vi "IETS_Tool_14_0805_bias_correct_neg_setpoints_ProbeStation.vi"() -> ()   [LabVIEW 2013]
doc: "I. Description:\nThis example demonstrates how to continuously acquire and generate data at the same time, synchronized with one another.\n\nII. Instructions for Running:\n1. Select the physical channel to correspond to where your signal is input on the DAQ device. Also, select the corresponding channel for where your signal is being generated.\n2. Enter the minimum and maximum voltage ranges.\nNote: For better accuracy try to match the input range to the expected voltage level of the measured signal.\n3. Set the sample rate of the acquisition.\nNote: The rate should be at least twice as fast as the maximum frequency component of the signal being acquired. \n6. Select the Rate for the generation\n7. Select what type of signal to generate and the amplitude.\nNote: This example requires two DMA channels to run. If your hardware does not support two DMA channels, you need to set the Data Transfer Mechanism property for the Analog Output Task to use \"Interrupts\". The Data Transfer Mechanism property is located in the DAQmx Channel Property hierarchy at:\n\nDAQmx Channel Property Node>>Analog Output>>General Properties>>Advanced>>Data Transfer and Memory>>Data Transfer Mechanism\n\nRefer to your device documentation to determine how many DMA channels are supported for your hardware.\n\nIII. Block Diagram Steps:\n1. Create an analog input voltage channel. Also, create an analog output voltage channel.\n2. Set the rate for the sample clock. Additionally, define the sample mode to be continuous. Also, set the sample clock rate for the signal generation.\n2a. Call the Get Terminal Name with Device Prefix VI. This will take a Task and a terminal and create a properly formatted device + terminal name to use as the source of the Trigger.\n3. Define the parameters for a Digital Edge Start Trigger. Set the Analog output to trigger off the AI Start Trigger. This is an internal trigger signal.\n4. Use the Basic Function Generator VI to create the signal to be generated.\n5. Call the Start VI to arm the two functions. Make sure the analog output is armed before the analog input. This will ensure both will start at the same time.\n6. Read the waveform data in a loop until the user hits the stop button or an error occurs. The Is Task Done? VI is used to check for errors in the Analog Output Task.\n7. Call the Clear VI to Clear the Task\n8. Use the popup dialog box to display an error if any.\n\nIV. I/O Connections Overview:\nMake sure your signal input/output terminals match the Physical Channel I/O controls."
uses:
  <vilib>/Utility/error.llb/DialogType.ctl
  <vilib>/DAQmx/write.llb/DAQmx Write (Analog 2D DBL NChan NSamp).vi
  <vilib>/DAQmx/read.llb/DAQmx Read (Analog 1D DBL NChan 1Samp).vi
  <vilib>/DAQmx/write.llb/DAQmx Write (Analog DBL 1Chan 1Samp).vi
  <vilib>/DAQmx/read.llb/DAQmx Read (Analog DBL 1Chan 1Samp).vi
  <vilib>/Analysis/baseanly.llb/Mean (DBL).vi
  <vilib>/DAQmx/write.llb/DAQmx Write (Analog 1D DBL NChan 1Samp).vi
  <vilib>/DAQmx/create/channels.llb/DAQmx Create Channel (AO-Voltage-Basic).vi
  <vilib>/DAQmx/create/channels.llb/DAQmx Create Channel (AI-Voltage-Basic).vi
  <vilib>/DAQmx/configure/timing.llb/DAQmx Timing (Sample Clock).vi
  <vilib>/DAQmx/configure/trigger.llb/DAQmx Start Trigger (Digital Edge).vi
  <vilib>/DAQmx/miscellaneous.llb/DAQmx Fill In Error Info.vi
  <vilib>/Utility/file.llb/Write To Spreadsheet File (DBL).vi
  pid/pid.llb/PID (DBL).vi
  pid/pid.llb/PID Output Rate Limiter (DBL).vi
  <vilib>/ptbypt/NI_PtbyPt.lvlib
  <resource>/objmgr/daqmx.rc
  <vilib>/Analysis/NI_AALBase.lvlib
panel:
  in  "Bias Offset Correct":dbl
  out "Bias Sweep":dbl[](graph)
  out "element":dbl
  out "mean":dbl format="%.6f"
  out "size(s)":i32
  out "Numeric":i32
  in  "PID":bool=TRUE caption="Step Z"
  in  "Tab Control":enum32{"PID Controller", "Tapping Controls"}(tab)=enum."Tapping Controls"
  in  "Proportional Gain":dbl=0.0001
  in  "Integral Gain":dbl=1e-07
  in  "Differential Gain":dbl=1e-05
  in  "Setpoint":dbl=0.1
  in  "Piezo Delta rate":dbl=1000.0
  in  "Min Current":dbl=0.002
  in  "Max Current":dbl=10.2
  in  "Ramp Rate":dbl=20.0
  in  "Make Contact":i32=1200
  in  "Break Contact":i32=500
  in  "Step Length":i32=100
  in  "Step Max":dbl=0.3
  in  "Step Min":dbl=0.05
  out "Tapping Stop":bool
  out "Case":i32
  in  "Contact Cycles":i32
  in  "Tapping":bool caption="Step Z"
  out "x/y":dbl
  out "Waveform Chart":dbl(graph)
  in  "Analog Ouyput 1":dbl(slide) min=-10.0 max=10.0 step=0.001 scale=-10.0..10.0
  in  "Manual Z":bool caption="Step Z"
  in  "Sweep Amplitude":dbl=1.0
  in  "Stop Sweep":bool
  out "Connections 2":string="AI0=Current\nAI1=Bias\nAI2=dI/dV\nAI3=d2I/dV2\nAI4=X-Axis\nAI5=Z-Axis\n"
  out "Connections":string="AO0=Bias\nAO1=Z-axis\nAO2=X-Axis\nAO3=NA"
  out "Save Indicator":bool
  in  "Z-Direction":bool caption="Step Z"
  in  "Update Bias":bool
  in  "Save IV":bool
  in  "Save Decay":bool
  in  "Sweep Bias":bool
  in  "Step Z":bool
  in  "Comment":string="Molecule=TP4\nGain=10nA\nBias Gain=div/1\nSweep Freq.=0.0008Hz\nRef. Bias=4mV\nRef. Freq=2.977kHz\nGain LIA1=2mV\nTC LIA1=1s\nGain LIA2=5mV\nTC LIA2=1s\nLIA1=EGG\nLIA2=SRS\nEGG is driving(possible 5mV offset)"
  in  "Filenumber":i32
  in  "DATA Filename":string="Data_"
  in  "Data Directory":path=path "E:/Research/Data"
  out "Current Decay":cluster{dbl[], dbl[]}(graph)
  out "d2I/dV2":cluster{dbl[], dbl[]}(graph)
  out "dI/dV":cluster{dbl[], dbl[]}(graph)
  out "IV":cluster{dbl[], dbl[]}(graph)
  in  "# Samples":i32=2000
  in  "Frequency (Hz)":dbl=1.0
  out "Measurement 2":cluster{i32, dbl, dbl[]}(graph) caption="Measurement"
  out "Actual Update Generation Rate 2":dbl=5000.0 caption="Actual Update Generation Rate" format="%0.2f"
  in  "stop 3":bool
  in  "Bias":dbl=0.1 caption="Bias Start Point" step=0.1 format="%_3g"
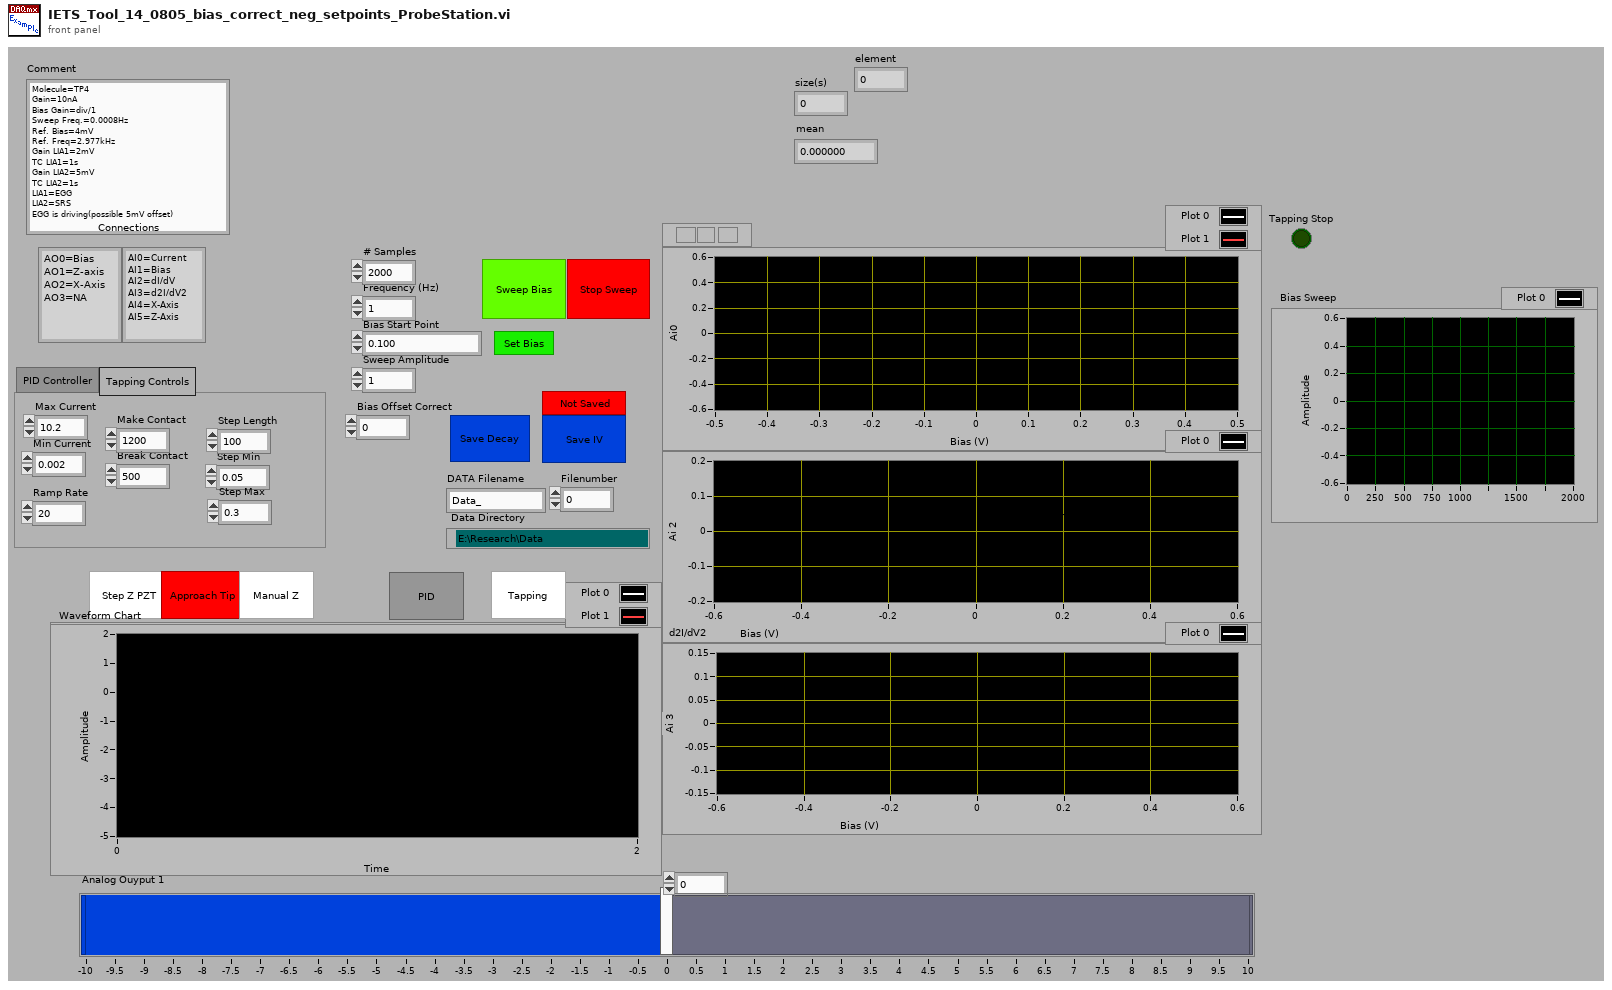
[diagram p1: front panel]
types:
  T1 = enum16{"open", "replace", "create", "open or create", "replace or create", "replace or create with confirmation"}
  T2 = typedef "DialogType.ctl" = u16
  T3 = cluster{"Proportional Gain":dbl, "Integral Gain ":dbl, "Differential Gain":dbl}
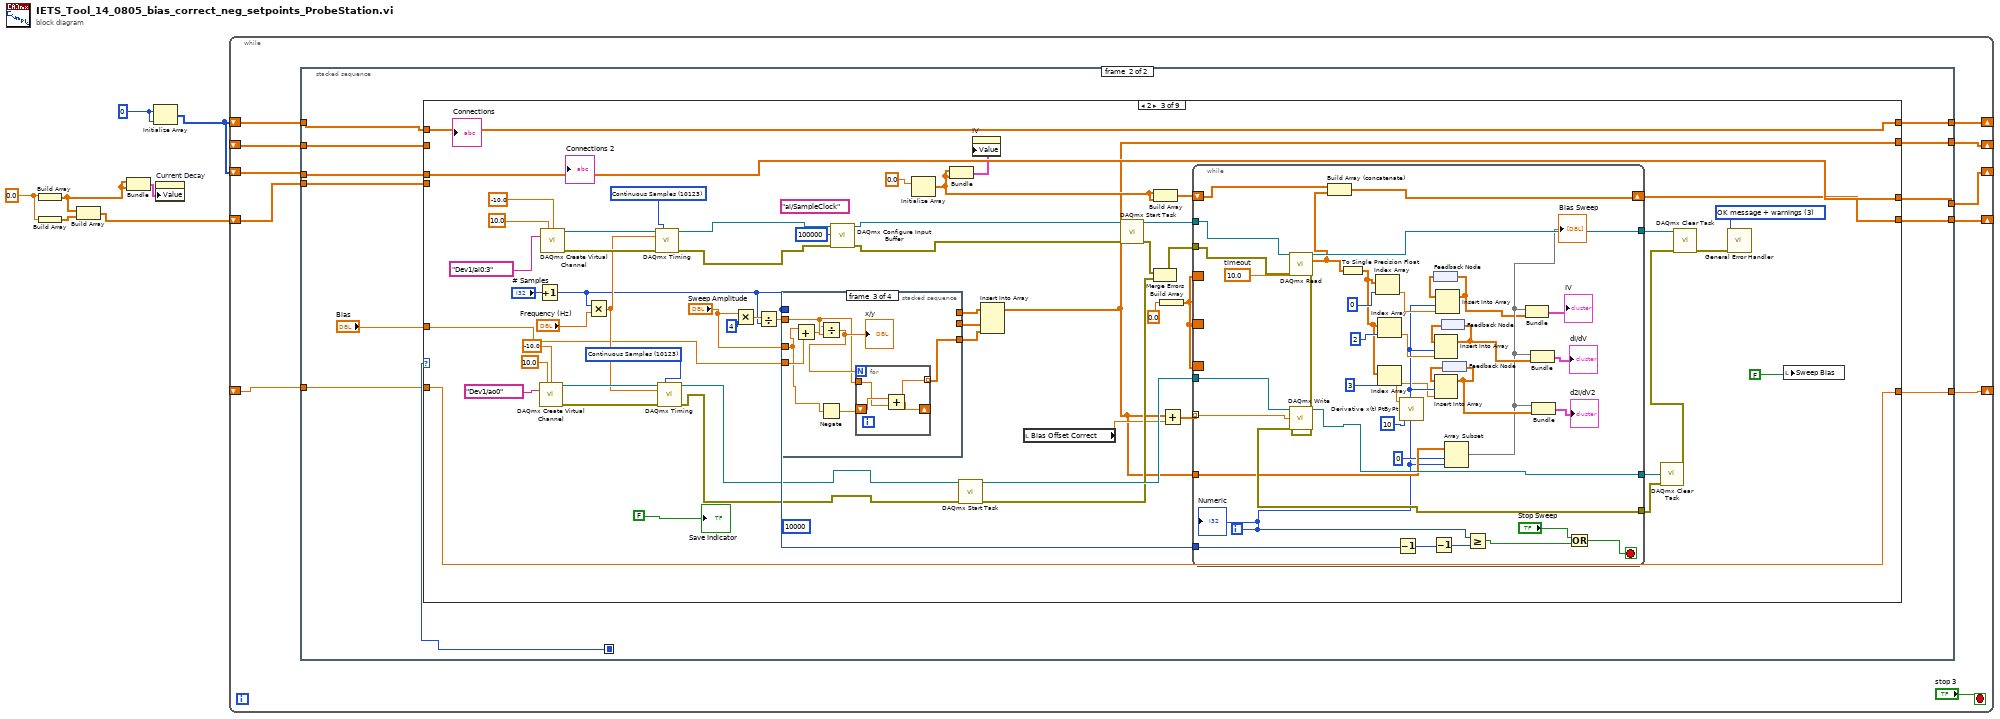
[diagram p0: block diagram]
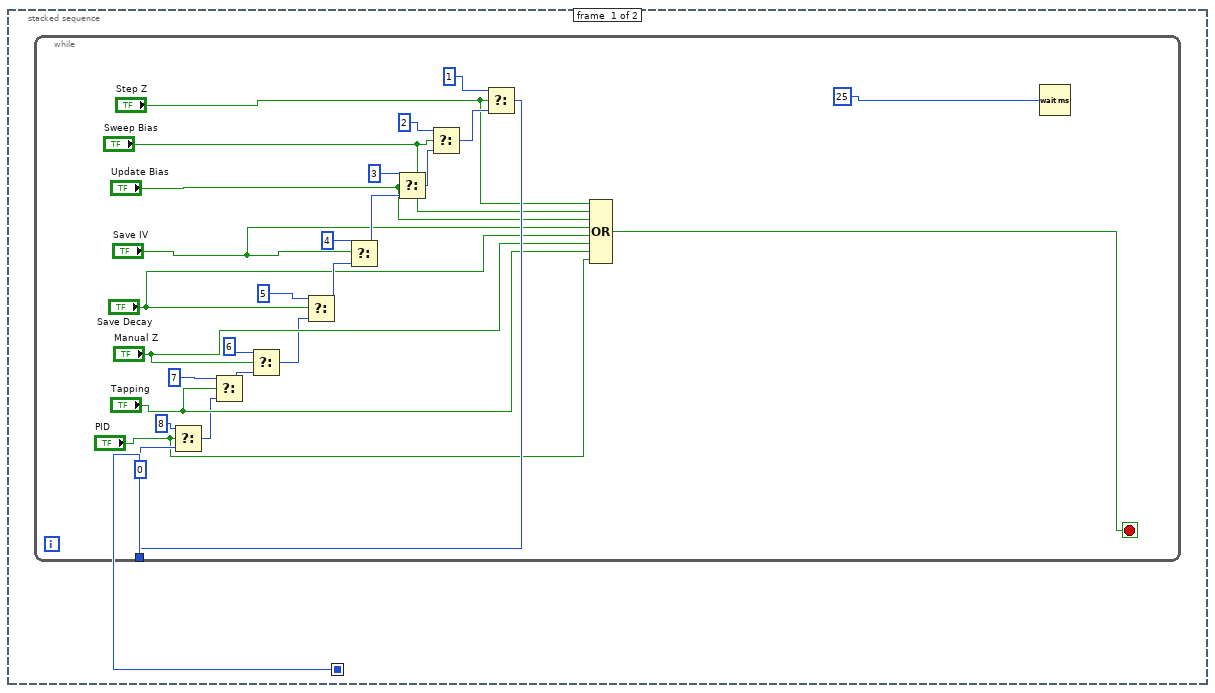
[diagram p2: hidden frame]
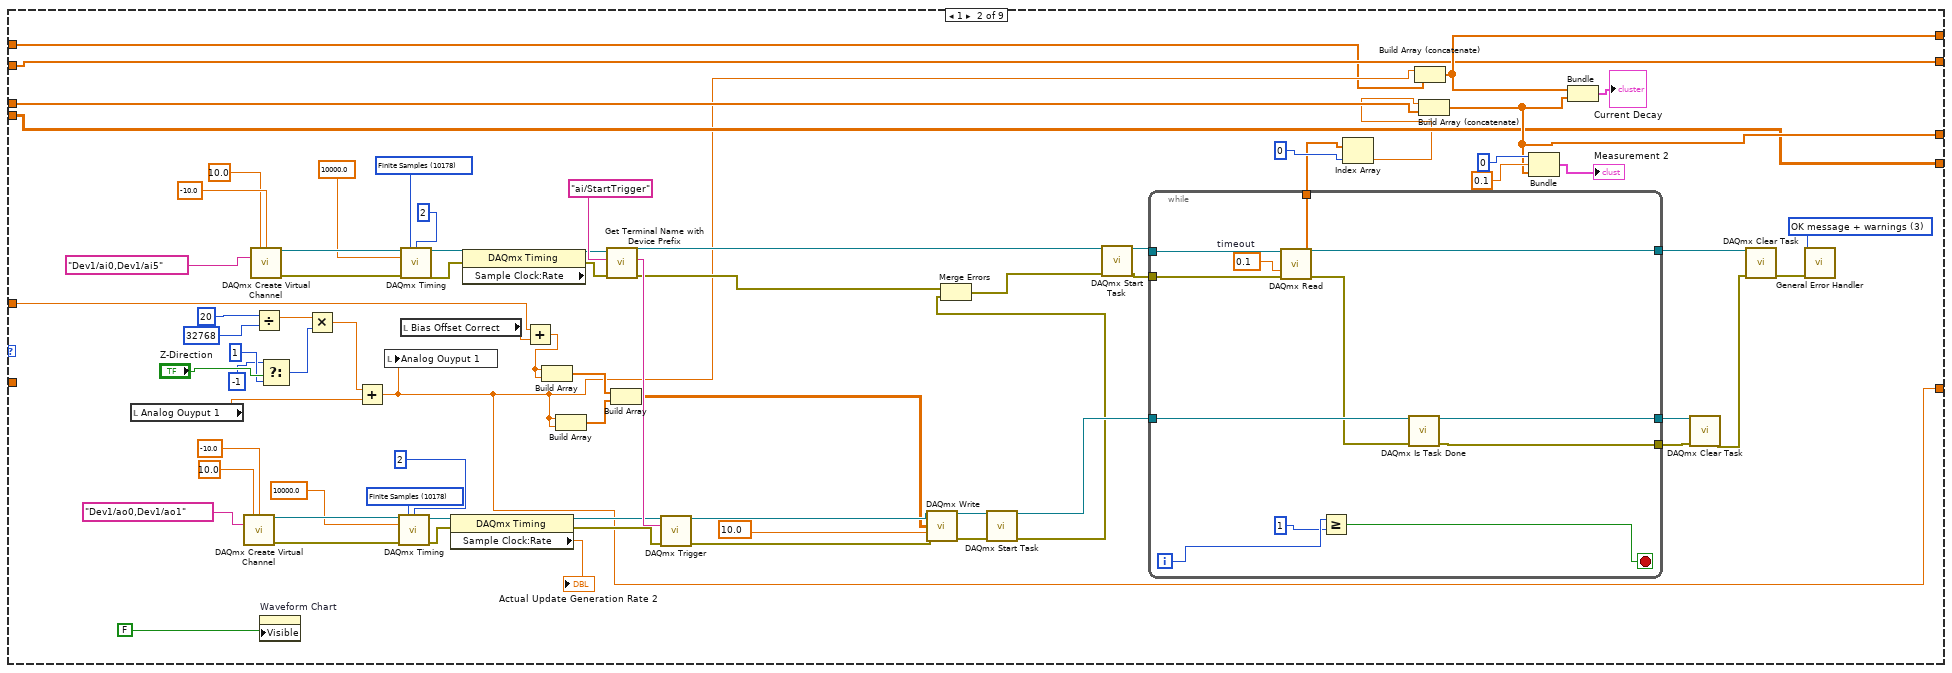
[diagram p4: hidden frame]
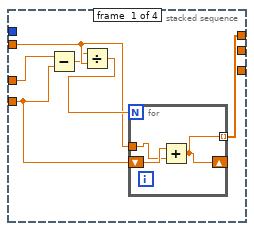
[diagram p5: hidden frame]
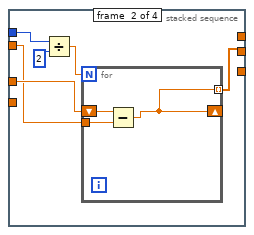
[diagram p6: hidden frame]
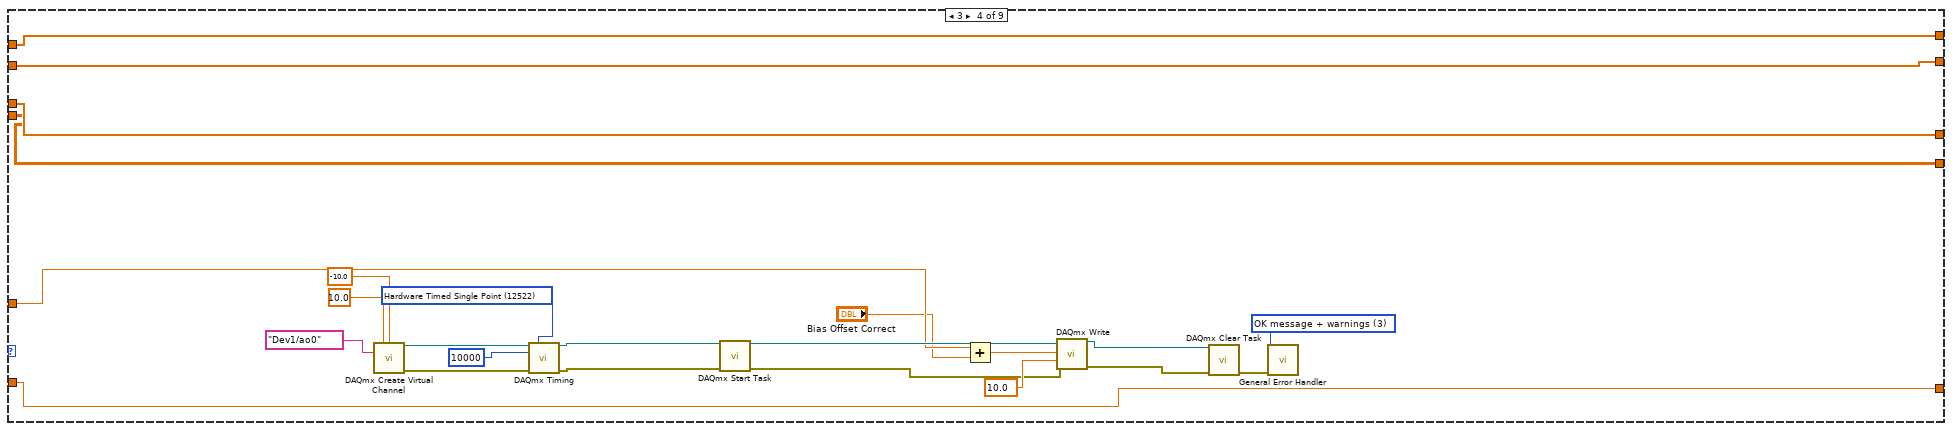
[diagram p8: hidden frame]
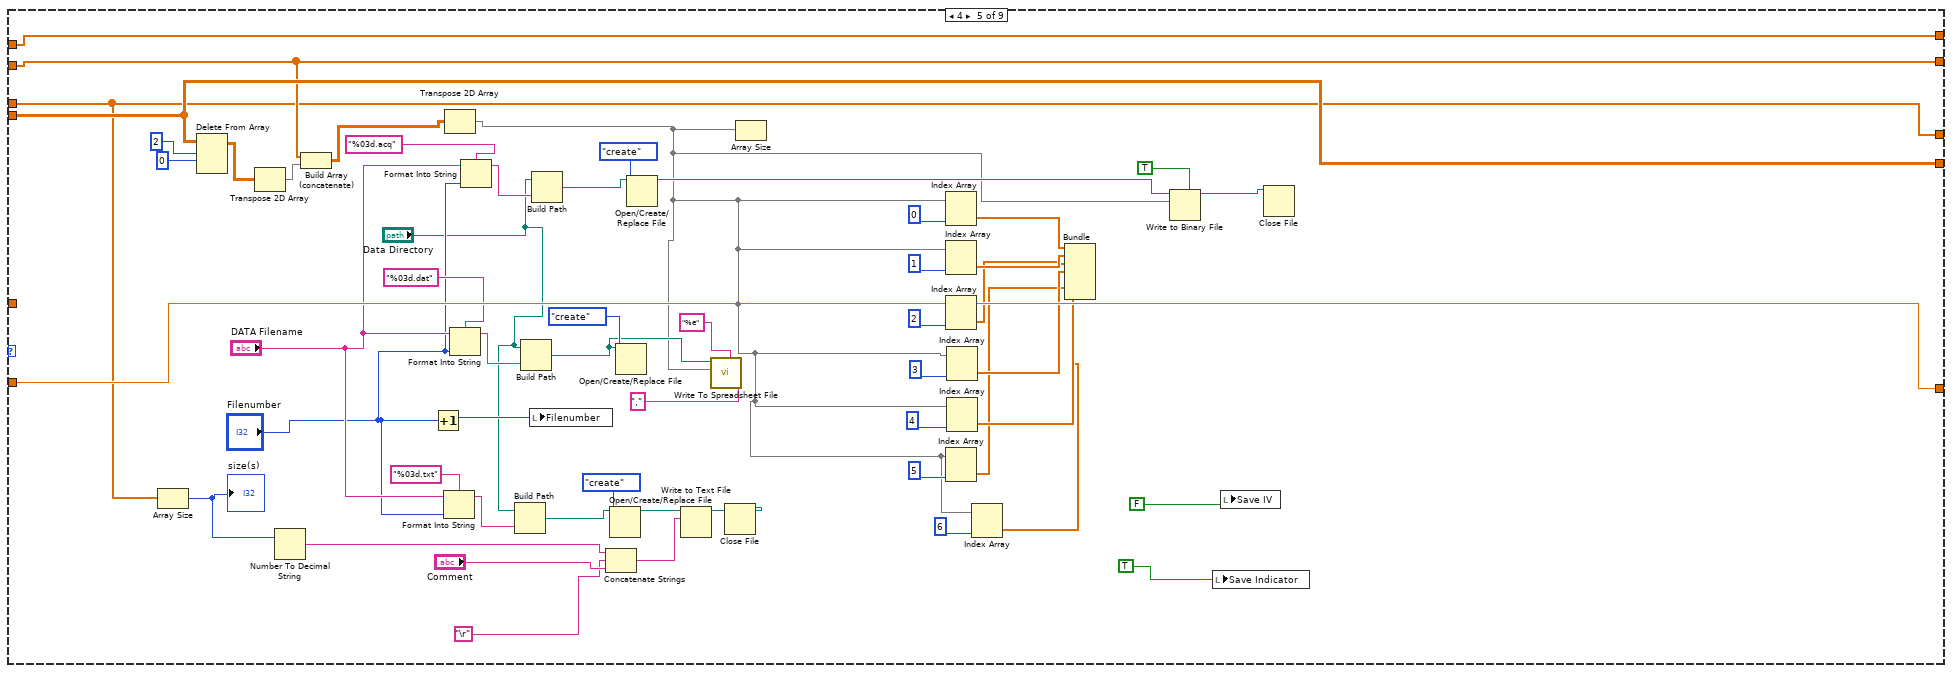
[diagram p9: hidden frame]
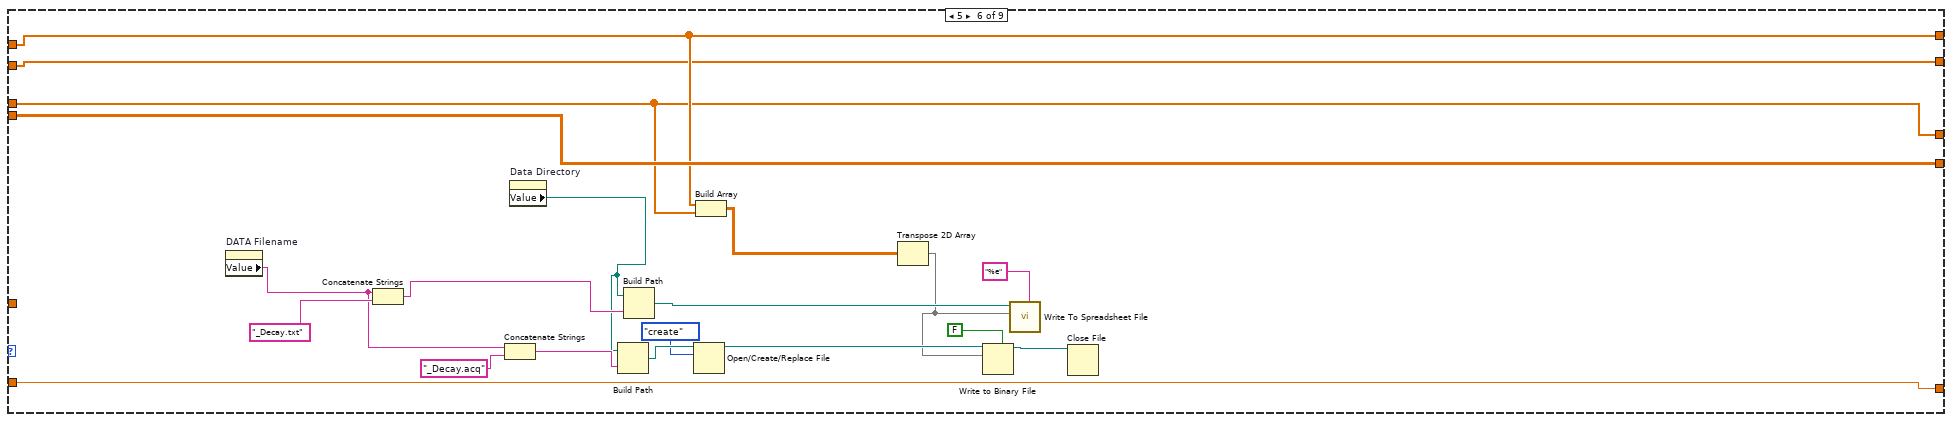
[diagram p10: hidden frame]
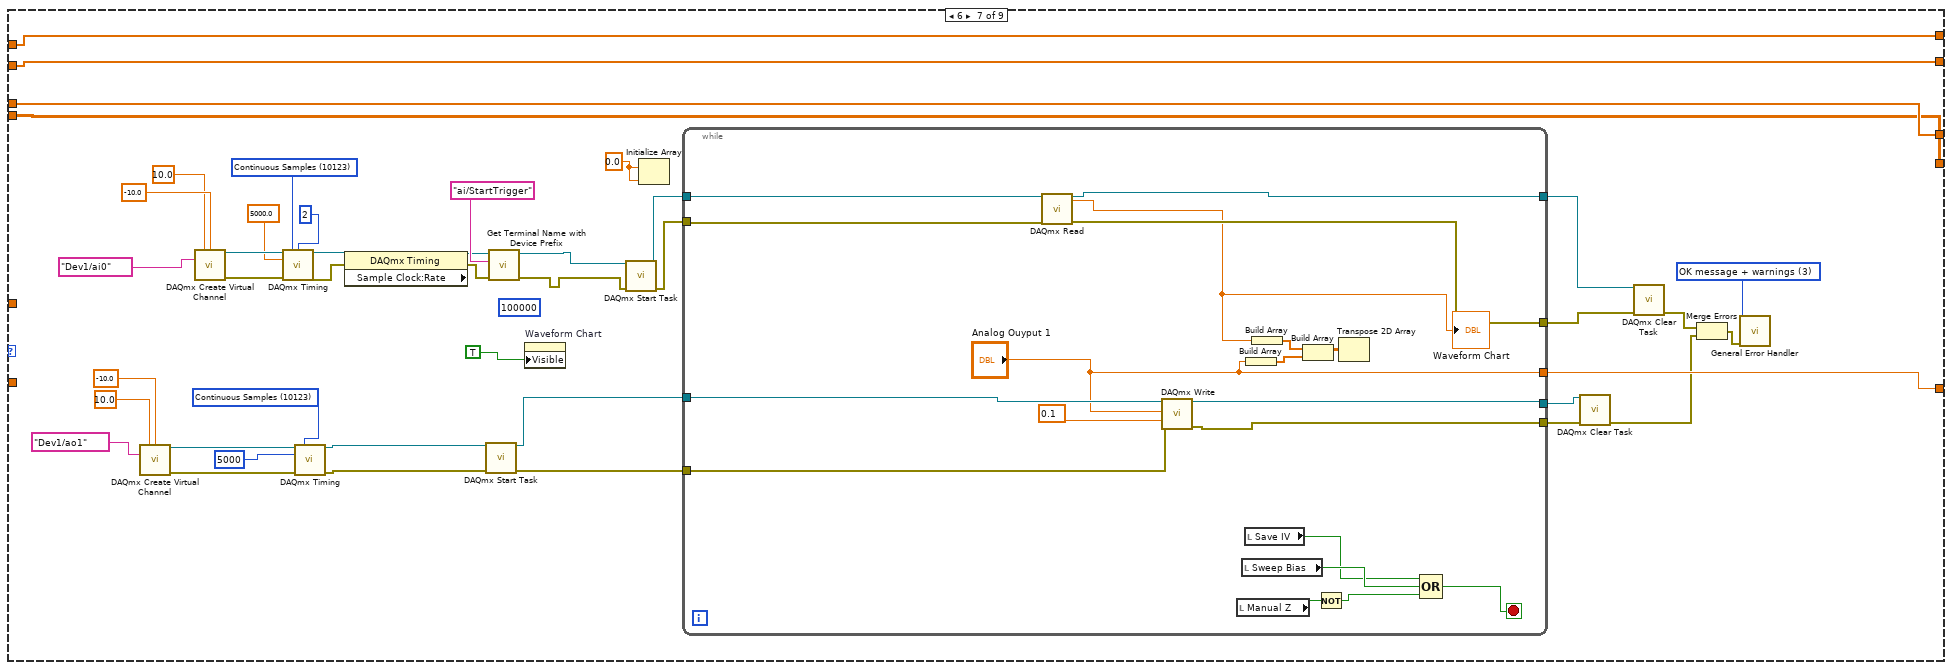
[diagram p11: hidden frame]
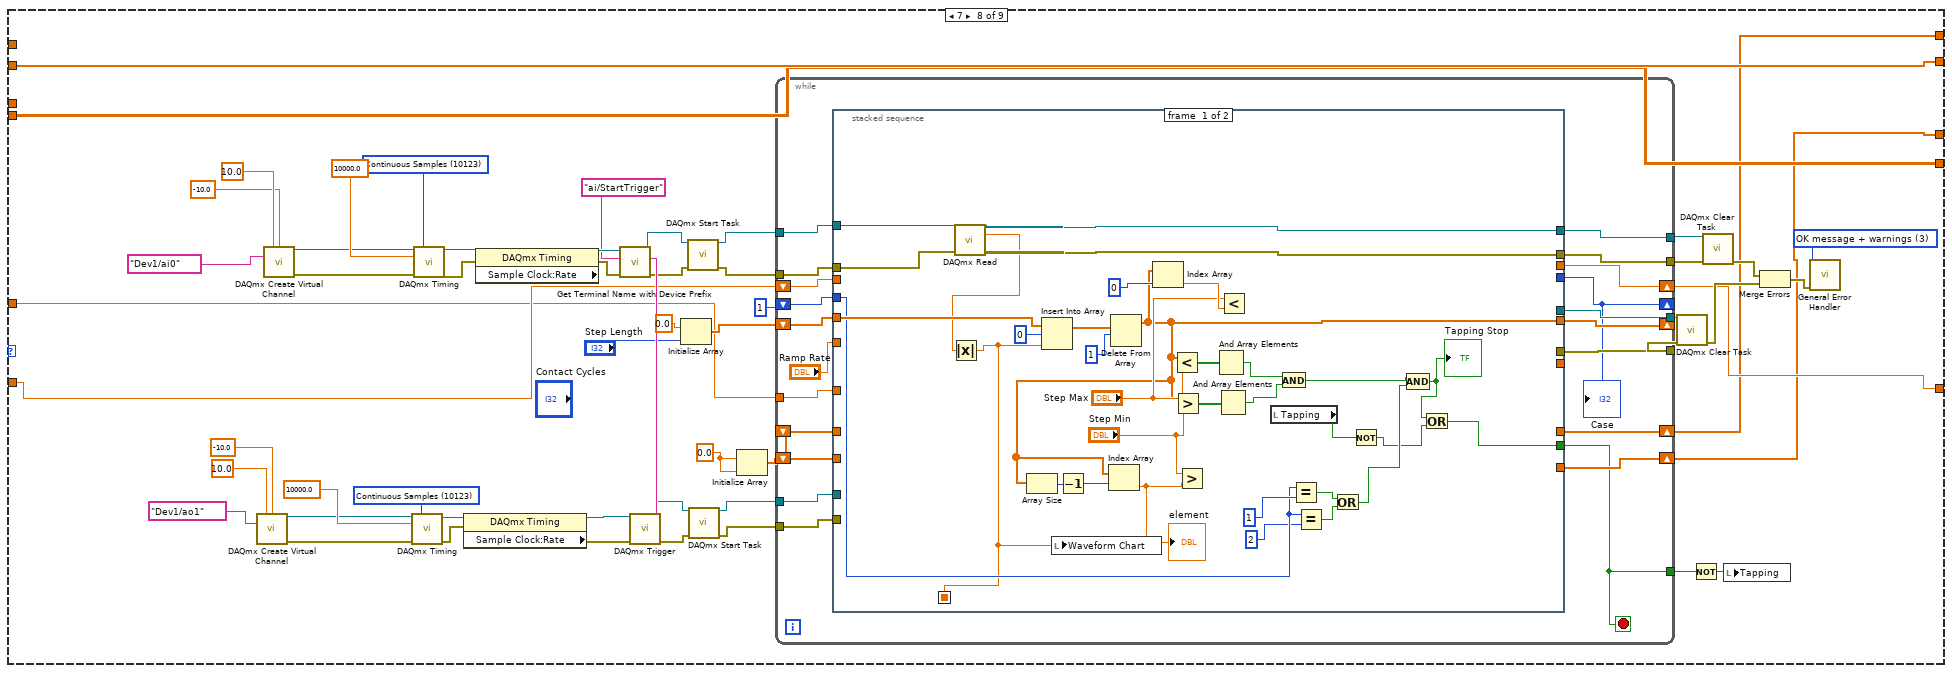
[diagram p12: hidden frame]
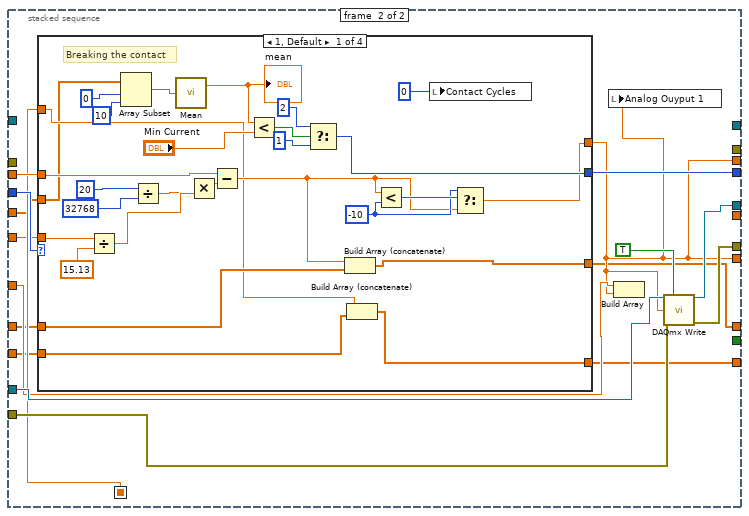
[diagram p13: hidden frame]
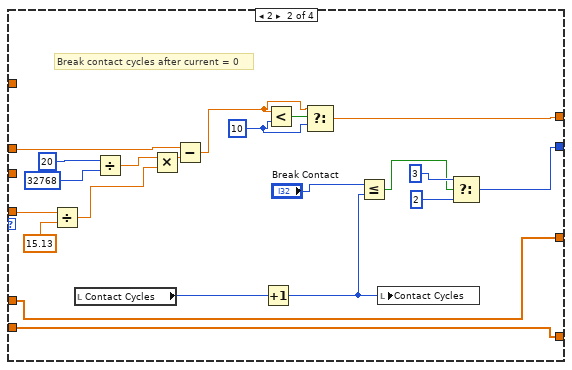
[diagram p14: hidden frame]
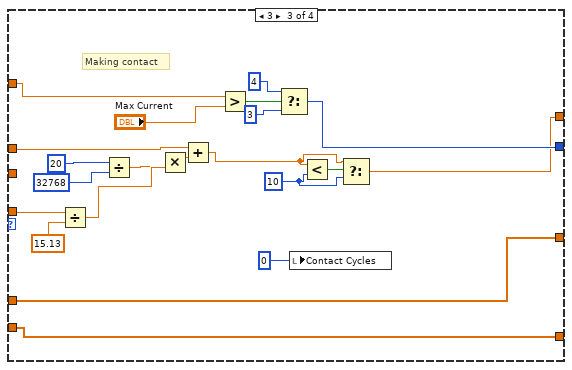
[diagram p15: hidden frame]
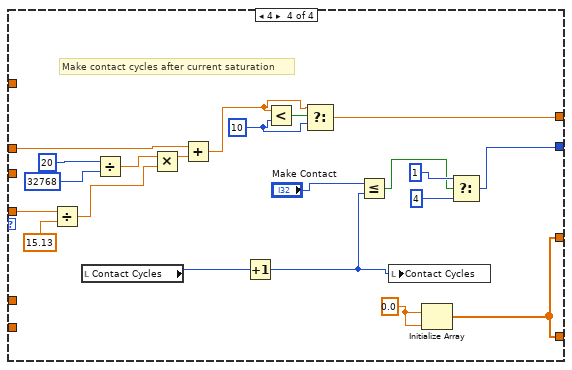
[diagram p16: hidden frame]
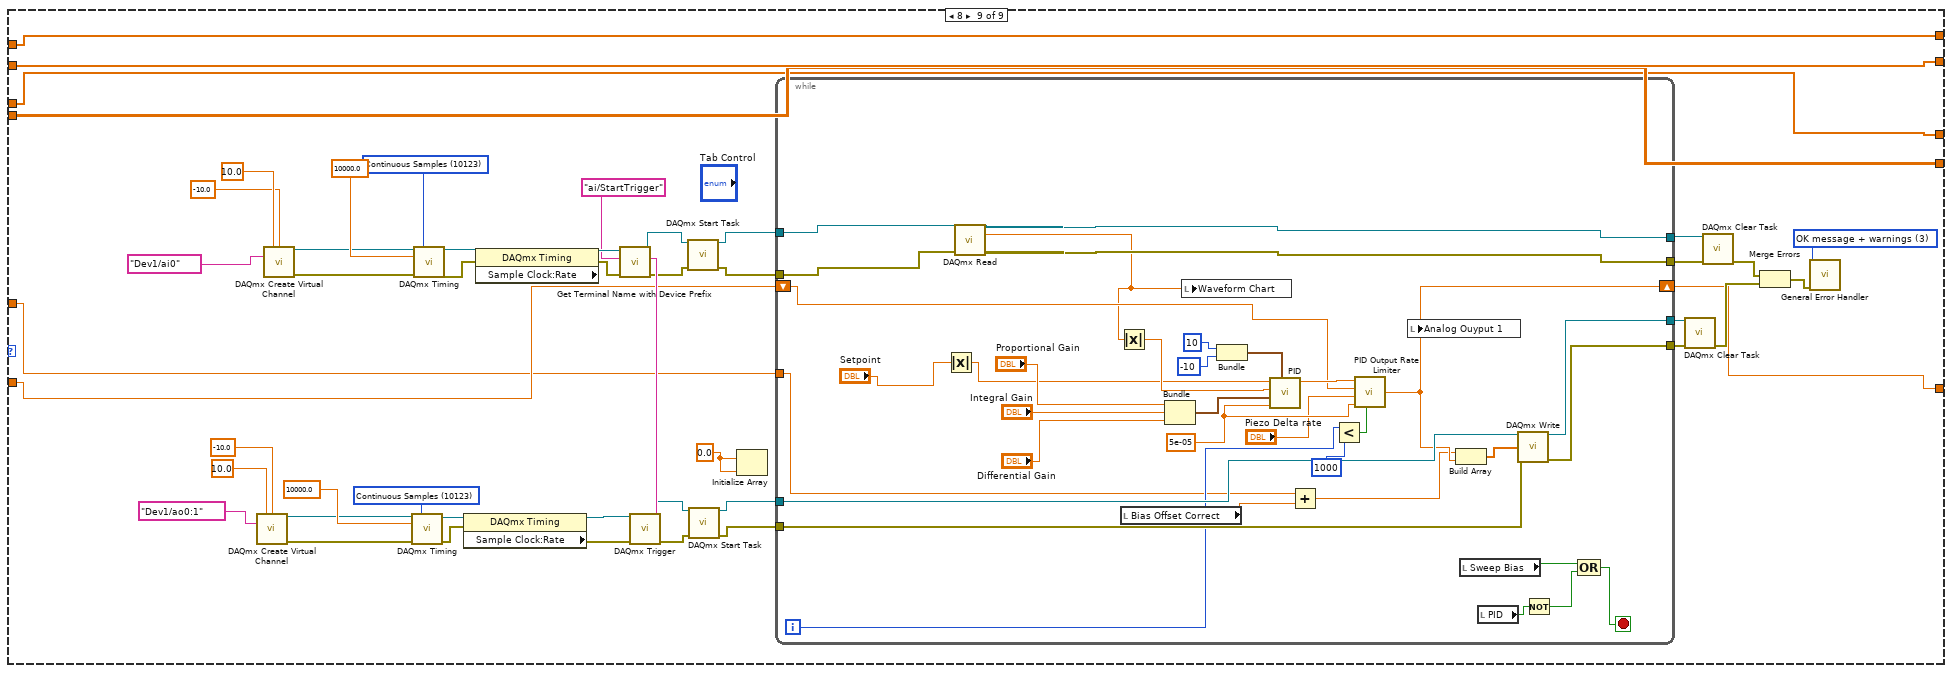
[diagram p17: hidden frame]
diagram:
  w2 = 0
  w7 = 0.0
  n1 = Build Array(w7) -> (w4:dbl[])
  n2 = Build Array(w7) -> (w6:dbl[])
  n3 = Build Array(w4, w6) -> (w5:dbl[][])
  n4 = Bundle(w4, w4) -> (w3:cluster{dbl[], dbl[]})  [unwired: 1 in]
  n5 = Initialize Array(w2, w2) -> (w1:i32[])
  n6 = property on="Current Decay" class="XYGraph (strict)"("Value"=w3) -> ()  [unwired: 2 in, 2 out]
  n7 = while {
    shift-right: [w16] -> _
    shift-left: w1 -> [w17]
    shift-right: [w14] -> _
    shift-left: w1 -> [w15]
    shift-right: [w12] -> _
    shift-left: _ -> [w13]
    shift-right: [w10] -> _
    shift-left: w5 -> [w11]
    shift-right: [w8] -> _
    shift-left: _ -> [w9]
    stop <- "stop 3" stop-if-true
    n8 = stacked-sequence {
      seq-local: [w19 _] -> [_ w58]
      tunnel: w17 -> [_ w57]
      tunnel: [_ w56] -> w16
      tunnel: w15 -> [_ w54]
      tunnel: [_ w53] -> w14
      tunnel: w13 -> [_ w52]
      tunnel: [_ w47] -> w12
      tunnel: w11 -> [_ w51]
      tunnel: [_ w50] -> w10
      tunnel: w9 -> [_ w49]
      tunnel: [_ w48] -> w8
      frame #0 {
        n9 = while {
          tunnel: [w37] -> w19
          stop <- w36 stop-if-true
          n10 = Select(t=8, s="PID", f=0) -> (s? t:f=w23:i32)
          n11 = Select(t=7, s="Tapping", f=w23) -> (s? t:f=w25:i32)
          n12 = Select(t=6, s="Manual Z", f=w25) -> (s? t:f=w26:i32)
          n13 = Select(t=5, s="Save Decay", f=w26) -> (s? t:f=w42:i32)
          n14 = Select(t=4, s="Save IV", f=w42) -> (s? t:f=w41:i32)
          n15 = Select(t=3, s="Update Bias", f=w41) -> (s? t:f=w39:i32)
          n16 = Select(t=2, s="Sweep Bias", f=w39) -> (s? t:f=w46:i32)
          n17 = Select(t=1, s="Step Z", f=w46) -> (s? t:f=w37:i32)
          n18 = Compound Arithmetic op=OR("Step Z", "Sweep Bias", "Update Bias", "Save IV", "Save Decay", "Manual Z", "Tapping", "PID") -> (w36:bool)
          n19 = Wait (ms)(milliseconds to wait=25) -> ()  [unwired: 1 out]
        }
      }
      frame #1 {
        n20 = case shown="2" w58 {
          tunnel: w57 -> [w63 w70 w191 w282 w302 w369 w414 _ w654]
          tunnel: [w63 w83 w191 w282 w302 w369 w414 w440 w654] -> w56
          tunnel: "Bias" -> [_ w66 w176 w276 _ _ _ w446 w653]
          tunnel: w54 -> [w62 w67 w188 w283 w349 w370 w416 _ w655]
          tunnel: [w62 w84 w188 w283 w349 w370 w416 w441 w655] -> w53
          tunnel: w52 -> [w61 _ w187 w281 w348 w371 _ w447 w662]
          tunnel: [w61 w68 w187 w281 w348 w371 w385 w442 w659] -> w47
          tunnel: w51 -> [w60 w81 _ w279 w328 w372 w413 w444 w660]
          tunnel: [w60 w81 w168 w279 w328 w372 w413 w444 w660] -> w50
          tunnel: [w59 w76 w151 w278 w326 w354 w415 w445 w661] -> w48
          tunnel: w49 -> [w59 w76 _ w278 w326 w354 w415 w445 w661]
          frame 0, Default {
          }
          frame 1 {
            w118 = T2 3 items=["no dialog", "OK message", "continue or stop message", "OK message + warnings", "continue/stop + warnings"] ("type of dialog (OK msg:1)")
            w130 = 10178 items=["Finite Samples"=10178, "Continuous Samples"=10123] ("sample mode")
            w135 = 10178 items=["Finite Samples"=10178, "Continuous Samples"=10123] ("sample mode")
            n21 = local read "Analog Ouyput 1"() -> (w71:dbl)
            n22 = call-poly <vilib>:"DAQmx Create Virtual Channel.vi"("maximum value"=10.0 ("maximum value 2"), "minimum value"=-10.0 ("minimum value 2"), "physical channels"=tag "Dev1/ao0,Dev1/ao1" ("physical channels 2")) -> ("task out"=w129:refnum<k21>, "error out"=w128:errorcluster)  [unwired: 11 in]
            n23 = call-poly <vilib>:"DAQmx Create Virtual Channel.vi"("maximum value"=10.0 ("Maximum Value 2"), "minimum value"=-10.0 ("Minimum Value 2"), "physical channels"=tag "Dev1/ai0,Dev1/ai5" ("Physical Channel 2")) -> ("task out"=w133:refnum<k21>, "error out"=w134:errorcluster)  [unwired: 11 in]
            n24 = Divide(x=20, y=32768) -> (x/y=w80:dbl)
            n25 = property on="Waveform Chart" class="WFChart (strict)"("Visible"=FALSE) -> ()  [unwired: 2 in, 2 out]
            n26 = Select(t=-1 ("f"), s="Z-Direction", f=1) -> (s? t:f=w78:i32)
            n27 = Multiply(x=w80, y=w78) -> (x*y=w79:dbl)
            n28 = Add(x=w79, y=w71) -> (x+y=w68:dbl)
            n29 = local write "Analog Ouyput 1"(w68) -> ()
            n30 = call-poly <vilib>:"DAQmx Timing.vi"("task/channels in"=w129, "sample mode"=w130, "samples per channel"=2, "rate"=10000.0 ("rate 2"), "error in"=w128) -> ("task out"=w113:refnum<k21>, "error out"=w112:errorcluster)  [unwired: 9 in]
            n31 = call-poly <vilib>:"DAQmx Timing.vi"("task/channels in"=w133, "sample mode"=w135, "samples per channel"=2, "rate"=10000.0 ("Rate 2"), "error in"=w134) -> ("task out"=w107:refnum<k21>, "error out"=w106:errorcluster)  [unwired: 9 in]
            n32 = local read "Bias Offset Correct"() -> (w65:dbl)
            n33 = property class="DAQmx Timing"(reference=w113, error in=w112) -> (reference out=w114:refnum<k21>, error out=w111:errorcluster, "Sample Clock:Rate"=→"Actual Update Generation Rate 2":dbl)
            n34 = property class="DAQmx Timing" props=["Sample Clock:Rate"](reference=w107, error in=w106) -> (reference out=w105:refnum<k21>, error out=w104:errorcluster)  [unwired: 1 out]
            n35 = Add(x=w66, y=w65) -> (x+y=w64:dbl)
            n36 = Build Array(w64, w64) -> (w91:dbl[])
            n37 = Build Array(w68, w68) -> (w90:dbl[])
            n38 = call "Get Terminal Name with Device Prefix.vi"("error in (no error)"=w104, "Local Terminal Name"="ai/StartTrigger" ("terminal"), "task/channels in"=w105) -> ("error out"=w110:errorcluster, "Terminal Name with Device Prefix"=w115:tag, "task out"=w95:refnum<k21>)  [unwired: 6 in]
            n39 = Build Array(w91, w90) -> (w89:dbl[][])
            n40 = call-poly <vilib>:"DAQmx Trigger.vi"("task/channels in"=w114, "source"=w115, "error in"=w111) -> ("task out"=w120:refnum<k21>, "error out"=w121:errorcluster)  [unwired: 11 in]
            n41 = call-poly <vilib>:"DAQmx Write.vi"("task/channels in"=w120, "data"=w89, "timeout"=10.0 ("Wirite Timeout"), "error in"=w121) -> ("task out"=w123:refnum<k21>, "error out"=w122:errorcluster)  [unwired: 9 in, 1 out]
            n42 = call <vilib>:"DAQmx Start Task.vi"("task/channels in"=w123, "error in"=w122) -> ("task out"=w127:refnum<k21>, "error out"=w109:errorcluster)  [unwired: 12 in]
            n43 = Merge Errors(w110, w109) -> (w97:errorcluster)
            n44 = call <vilib>:"DAQmx Start Task.vi"("task/channels in"=w95, "error in"=w97) -> ("task out"=w94:refnum<k21>, "error out"=w96:errorcluster)  [unwired: 12 in]
            n45 = while {
              tunnel: [w150] -> w136
              tunnel: w127 -> [w149]
              tunnel: [w148] -> w126
              tunnel: w94 -> [w139]
              tunnel: [w147] -> w103
              tunnel: [w144] -> w87
              tunnel: w96 -> [w140]
              i -> [w143]
              stop <- w141 stop-if-true
              w146 = 0.1  # timeout
              n46 = call-poly <vilib>:"DAQmx Read.vi"("task/channels in"=w139, "timeout"=w146, "error in"=w140) -> ("task out"=w150:refnum<k21>, "data"=w144:dbl[], "error out"=w145:errorcluster)  [unwired: 10 in]
              n47 = Greater Or Equal?(x=w143, y=1) -> (x >= y?=w141:bool)
              n48 = call <vilib>:"DAQmx Is Task Done.vi"("task/channels in"=w149, "error in"=w145) -> ("task out"=w148:refnum<k21>, "error out"=w147:errorcluster)  [unwired: 11 in, 1 out]
            }
            n49 = Index Array(array=w87, index=0) -> (element=w69:dbl)
            n50 = Build Array (concatenate)(w68, w67) -> (w84:dbl[])
            n51 = Build Array (concatenate)(w69, w70) -> (w83:dbl[])
            n52 = Bundle(0, 0.1, w83) -> (→"Measurement 2":cluster{i32, dbl, dbl[]})  [unwired: 1 in]
            n53 = Bundle(w84, w83) -> (→"Current Decay":cluster{dbl[], dbl[]})  [unwired: 1 in]
            n54 = call <vilib>:"DAQmx Clear Task.vi"("task in"=w126, "error in"=w103) -> ("error out"=w102:errorcluster)  [unwired: 13 in]
            n55 = call <vilib>:"DAQmx Clear Task.vi"("task in"=w136, "error in"=w102) -> ("error out"=w101:errorcluster)  [unwired: 13 in]
            n56 = call <vilib>:"General Error Handler.vi"("type of dialog (OK msg:1)"=w118, "error in (no error)"=w101) -> ()  [unwired: 9 in, 5 out]
          }
          frame 2 {
            (unwired) 10000
            w185 = 10123 items=["Finite Samples"=10178, "Continuous Samples"=10123, "Hardware Timed Single Point"=12522] ("sample mode")
            w186 = 10123 items=["Finite Samples"=10178, "Continuous Samples"=10123, "Hardware Timed Single Point"=12522] ("sample mode")
            (unwired) "ai/SampleClock" ("terminal")
            w196 = T2 3 items=["no dialog", "OK message", "continue or stop message", "OK message + warnings", "continue/stop + warnings"] ("type of dialog (OK msg:1)")
            n57 = Increment(x="# Samples") -> (x+1=w166:i32)
            n58 = call-poly <vilib>:"DAQmx Create Virtual Channel.vi"("maximum value"=10.0, "minimum value"=-10.0, "physical channels"=tag "Dev1/ao0") -> ("task out"=w199:refnum<k21>, "error out"=w198:errorcluster)  [unwired: 11 in]
            n59 = call-poly <vilib>:"DAQmx Create Virtual Channel.vi"("maximum value"=10.0 ("Maximum Value"), "minimum value"=-10.0 ("Minimum Value"), "physical channels"=tag "Dev1/ai0:3" ("Physical Channel")) -> ("task out"=w203:refnum<k21>, "error out"=w204:errorcluster)  [unwired: 11 in]
            n60 = Multiply(x=w166, y="Frequency (Hz)") -> (x*y=w190:dbl)
            n61 = call-poly <vilib>:"DAQmx Timing.vi"("task/channels in"=w203, "sample mode"=w185, "rate"=w190, "error in"=w204) -> ("task out"=w160:refnum<k21>, "error out"=w158:errorcluster)  [unwired: 10 in]
            n62 = call-poly <vilib>:"DAQmx Timing.vi"("task/channels in"=w199, "sample mode"=w186, "rate"=w190, "error in"=w198) -> ("task out"=w155:refnum<k21>, "error out"=w154:errorcluster)  [unwired: 10 in]
            n63 = Multiply(x="Sweep Amplitude", y=4) -> (x*y=w174:dbl)
            n64 = Divide(x=w174, y=w166) -> (x/y=w173:dbl)
            n65 = stacked-sequence {
              tunnel: "Sweep Amplitude" -> [w252 w258 w266 _]
              tunnel: w176 -> [w250 _ w270 _]
              tunnel: w173 -> [w248 w257 w268 _]
              tunnel: [w249 _ _ _] -> w172
              tunnel: w166 -> [_ w261 _ _]
              tunnel: [_ w256 _ _] -> w171
              tunnel: [_ _ w269 _] -> w170
              frame #0 {
                n66 = Subtract(x=w252, y=w250) -> (x-y=w247:dbl)
                n67 = Divide(x=w247, y=w248) -> (x/y=w251:dbl)
                n68 = for {
                  N: w251 -> [_]
                  tunnel: w248 -> [w254]
                  shift-right: [w253] -> _
                  shift-left: w250 -> [w255]
                  tunnel: [w253] -> w249 mode=indexing
                  n69 = Add(x=w255, y=w254) -> (x+y=w253:dbl)
                }
              }
              frame #1 {
                n70 = Divide(x=w261, y=2) -> (x/y=w259:dbl)
                n71 = for {
                  N: w259 -> [_]
                  tunnel: w257 -> [w263]
                  shift-right: [w262] -> _
                  shift-left: w258 -> [w264]
                  tunnel: [w262] -> w256 mode=indexing
                  n72 = Subtract(x=w264, y=w263) -> (x-y=w262:dbl)
                }
              }
              frame #2 {
                n73 = Add(x=w266, y=w270) -> (x+y=w267:dbl)
                n74 = Divide(x=w267, y=w268) -> (x/y=w271:dbl)
                "x/y" <- w271
                n75 = Negate(x=w266) -> (-x=w265:dbl)
                n76 = for {
                  N: w271 -> [_]
                  tunnel: w268 -> [w273]
                  shift-right: [w272] -> _
                  shift-left: w265 -> [w274]
                  tunnel: [w272] -> w269 mode=indexing
                  n77 = Add(x=w274, y=w273) -> (x+y=w272:dbl)
                }
              }
              frame #3 {
              }
            }
            n78 = call <vilib>:"DAQmx Configure Input Buffer.vi"("task/channels in"=w160, "buffer size (in samples per channel)"=100000, "error in"=w158) -> ("task out"=w159:refnum<k21>, "error out"=w157:errorcluster)  [unwired: 11 in]
            n79 = Initialize Array(0.0) -> (w165:dbl[])  [unwired: 1 in]
            n80 = Bundle(w165, w165) -> (w164:cluster{dbl[], dbl[]})  [unwired: 1 in]
            n81 = call <vilib>:"DAQmx Start Task.vi"("task/channels in"=w155, "error in"=w154) -> ("task out"=w184:refnum<k21>, "error out"=w180:errorcluster)  [unwired: 12 in]
            n82 = property on="IV" class="XYGraph (strict)"("Value"=w164) -> ()  [unwired: 2 in, 2 out]
            n83 = Insert Into Array(array=w172, new element #1=w171, new element #2=w170) -> (w151:dbl[])  [unwired: 1 in]
            n84 = local read "Bias Offset Correct"() -> (w152:dbl)
            n85 = call <vilib>:"DAQmx Start Task.vi"("task/channels in"=w159, "error in"=w157) -> ("task out"=w182:refnum<k21>, "error out"=w181:errorcluster)  [unwired: 12 in]
            n86 = Merge Errors(w181, w180) -> (w183:errorcluster)
            n87 = Build Array(w165, w165) -> (w167:dbl[][])
            n88 = Build Array(0.0) -> (w162:dbl[])
            n89 = Add(x=w151, y=w152) -> (x+y=w153:dbl[])
            n90 = while {
              tunnel: [w238] -> w205
              tunnel: [w241] -> w197
              tunnel: [w240] -> w194
              tunnel: w166 -> [w214]
              tunnel: w153 -> [w219] mode=indexing
              tunnel: w184 -> [w243]
              tunnel: w182 -> [w246]
              tunnel: w183 -> [w245]
              shift-right: [w220] -> w168
              shift-left: w167 -> [w239]
              tunnel: w151 -> [w236]
              border: w162 -> [_]
              border: w162 -> [_]
              border: w162 -> [_]
              i -> [w215]
              stop <- w216 stop-if-true
              w242 = 10.0  # timeout
              n91 = call-poly <vilib>:"DAQmx Read.vi"("task/channels in"=w246, "timeout"=w242, "error in"=w245) -> ("task out"=w238:refnum<k21>, "data"=w222:dbl[], "error out"=w244:errorcluster)  [unwired: 10 in]
              n92 = call-poly <vilib>:"DAQmx Write.vi"("task/channels in"=w243, "data"=w219, "error in"=w244) -> ("task out"=w241:refnum<k21>, "error out"=w240:errorcluster)  [unwired: 10 in, 1 out]
              n93 = Build Array (concatenate)(w239, w222) -> (w220:dbl[][])
              n94 = To Single Precision Float(number=w222) -> (single precision float=w221:sgl[])
              n95 = Index Array(array=w221, index=0) -> (element=w234:sgl)
              n96 = Index Array(array=w221, index=2) -> (element=w230:sgl)
              n97 = Index Array(array=w221, index=3) -> (element=w210:sgl)
              n98 = Decrement(x=w214) -> (x-1=w212:i32)
              n99 = call <vilib>:"Derivative x(t) PtByPt.vi"("dt"=10, "x"=w210) -> ()  [unwired: 2 in, 2 out]
              n100 = Decrement(x=w212) -> (x-1=w213:i32)
              n101 = feedback #1() -> (w233:dbl[])
              n102 = Insert Into Array(array=w233, index=w215, new element=w234) -> (w208:dbl[])
              n103 = feedback-in #1(w208) -> ()
              n104 = feedback #2() -> (w229:dbl[])
              n105 = Insert Into Array(array=w229, index=w215, new element=w230) -> (w227:dbl[])
              n106 = feedback-in #2(w227) -> ()
              n107 = feedback #3() -> (w228:dbl[])
              n108 = Insert Into Array(array=w228, index=w215, new element=w210) -> (w226:dbl[])
              n109 = feedback-in #3(w226) -> ()
              n110 = Array Subset(array=w236, index=0, length=w215) -> (w209:dbl[])
              "Bias Sweep" <- w209
              n111 = Greater Or Equal?(x=w215, y=w213) -> (x >= y?=w217:bool)
              n112 = Bundle(w209, w208) -> (→"IV":cluster{dbl[], dbl[]})  [unwired: 1 in]
              n113 = Bundle(w209, w227) -> (→"dI/dV":cluster{dbl[], dbl[]})  [unwired: 1 in]
              n114 = Bundle(w209, w226) -> (→"d2I/dV2":cluster{dbl[], dbl[]})  [unwired: 1 in]
              n115 = Or(x="Stop Sweep", y=w217) -> (x .or. y?=w216:bool)
              "Numeric" <- w215
            }
            n116 = call <vilib>:"DAQmx Clear Task.vi"("task in"=w197, "error in"=w194) -> ("error out"=w193:errorcluster)  [unwired: 13 in]
            n117 = call <vilib>:"DAQmx Clear Task.vi"("task in"=w205, "error in"=w193) -> ("error out"=w192:errorcluster)  [unwired: 13 in]
            n118 = call <vilib>:"General Error Handler.vi"("type of dialog (OK msg:1)"=w196, "error in (no error)"=w192) -> ()  [unwired: 9 in, 5 out]
            n119 = local write "Sweep Bias"(FALSE) -> ()
            "Save Indicator" <- FALSE
          }
          frame 3 {
            w287 = T2 3 items=["no dialog", "OK message", "continue or stop message", "OK message + warnings", "continue/stop + warnings"] ("type of dialog (OK msg:1)")
            w292 = 12522 items=["Finite Samples"=10178, "Continuous Samples"=10123, "Hardware Timed Single Point"=12522] ("sample mode")
            n120 = call-poly <vilib>:"DAQmx Create Virtual Channel.vi"("maximum value"=10.0 ("maximum value 2"), "minimum value"=-10.0 ("minimum value 2"), "physical channels"=tag "Dev1/ao0" ("physical channels 2")) -> ("task out"=w295:refnum<k21>, "error out"=w294:errorcluster)  [unwired: 11 in]
            n121 = call-poly <vilib>:"DAQmx Timing.vi"("task/channels in"=w295, "sample mode"=w292, "rate"=10000, "error in"=w294) -> ("task out"=w291:refnum<k21>, "error out"=w290:errorcluster)  [unwired: 10 in]
            n122 = call <vilib>:"DAQmx Start Task.vi"("task/channels in"=w291, "error in"=w290) -> ("task out"=w289:refnum<k21>, "error out"=w288:errorcluster)  [unwired: 12 in]
            n123 = Add(x=w276, y="Bias Offset Correct") -> (x+y=w277:dbl)
            n124 = call-poly <vilib>:"DAQmx Write.vi"("task/channels in"=w289, "data"=w277, "timeout"=10.0 ("Wirite Timeout"), "error in"=w288) -> ("task out"=w285:refnum<k21>, "error out"=w284:errorcluster)  [unwired: 9 in, 1 out]
            n125 = call <vilib>:"DAQmx Clear Task.vi"("task in"=w285, "error in"=w284) -> ("error out"=w286:errorcluster)  [unwired: 13 in]
            n126 = call <vilib>:"General Error Handler.vi"("type of dialog (OK msg:1)"=w287, "error in (no error)"=w286) -> ()  [unwired: 9 in, 5 out]
          }
          frame 4 {
            n127 = Array Size(array=w302) -> (size(s)=w301:i32)
            "size(s)" <- w301
            n128 = Delete From Array(array=w328, length=2, index (row)=0) -> (array with subset deleted=w325:dbl[][])  [unwired: 1 in, 1 out]
            n129 = Transpose 2D Array(2D array=w325) -> (transposed array=w324:dbl[][])
            n130 = Number To Decimal String(number=w301) -> (decimal integer string=w300:string)  [unwired: 1 in]
            n131 = Build Array (concatenate)(w326, w324) -> (w306:dbl[][])
            n132 = Increment(x="Filenumber") -> (x+1=w351:i32)
            n133 = Format Into String(format string="%03d.txt", initial string="DATA Filename", "Filenumber") -> (resulting string=w339:string)  [unwired: 1 in, 1 out]
            n134 = Transpose 2D Array(2D array=w306) -> (transposed array=w305:dbl[][])
            n135 = Format Into String(format string="%03d.dat", initial string="DATA Filename", "Filenumber") -> (resulting string=w353:string)  [unwired: 1 in, 1 out]
            n136 = Format Into String(format string="%03d.acq", initial string="DATA Filename", "Filenumber") -> (resulting string=w346:string)  [unwired: 1 in, 1 out]
            n137 = Build Path(base path="Data Directory", name or relative path=w339) -> (appended path=w337:path)
            n138 = Build Path(base path="Data Directory", name or relative path=w353) -> (appended path=w350:path)
            n139 = local write "Filenumber"(w351) -> ()
            n140 = Build Path(base path="Data Directory", name or relative path=w346) -> (appended path=w344:path)
            n141 = Concatenate Strings(w300, "\r", "Comment") -> (w322:string)
            n142 = Open/Create/Replace File(file path (use dialog)=w337, operation (0:open)=T1."create") -> (refnum out=w332:refnum<file>)  [unwired: 4 in, 2 out]
            n143 = Open/Create/Replace File(file path (use dialog)=w350, operation (0:open)=T1."create") -> ()  [unwired: 4 in, 3 out]
            n144 = Open/Create/Replace File(file path (use dialog)=w344, operation (0:open)=T1."create") -> (refnum out=w343:refnum<file>)  [unwired: 4 in, 2 out]
            n145 = Write to Text File(file (use dialog)=w332, text=w322) -> (refnum out=w331:refnum<file>)  [unwired: 2 in, 2 out]
            n146 = call-poly <vilib>:"Write To Spreadsheet File.vi"("delimiter (\\t)"=",", "format (%.3f)"="%e", "2D data"=w305, "file path (dialog if empty)"=w350) -> ()  [unwired: 4 in, 1 out]
            n147 = Close File(refnum=w331) -> ()  [unwired: 1 in, 2 out]
            n148 = Array Size(array=w305) -> ()  [unwired: 1 out]
            n149 = Index Array(array=w305, index (col)=0) -> (element=w314:dbl[])  [unwired: 1 in]
            n150 = Index Array(array=w305, index (col)=1) -> (element=w313:dbl[])  [unwired: 1 in]
            n151 = Index Array(array=w305, index (col)=2) -> (element=w312:dbl[])  [unwired: 1 in]
            n152 = Index Array(array=w305, index (col)=5) -> (element=w309:dbl[])  [unwired: 1 in]
            n153 = Index Array(array=w305, index (col)=3) -> (element=w311:dbl[])  [unwired: 1 in]
            n154 = Index Array(array=w305, index (col)=4) -> (element=w310:dbl[])  [unwired: 1 in]
            n155 = Index Array(array=w305, index (col)=6) -> (element=w308:dbl[])  [unwired: 1 in]
            n156 = Bundle(w314, w313, w312, w311, w310, w309, w308) -> ()  [unwired: 1 in, 1 out]
            n157 = Write to Binary File(file (use dialog)=w343, data=w305, 5:TRUE ("prepend array or string size? (T)")) -> (refnum out=w341:refnum<file>)  [unwired: 3 in, 2 out]
            n158 = local write "Save Indicator"(TRUE) -> ()
            n159 = local write "Save IV"(FALSE) -> ()
            n160 = Close File(refnum=w341) -> ()  [unwired: 1 in, 2 out]
          }
          frame 5 {
            n161 = property on="DATA Filename" class="Str"() -> ("Value"=w364:string)  [unwired: 2 in, 2 out]
            n162 = Concatenate Strings(w364, "_Decay.txt") -> (w368:string)
            n163 = Concatenate Strings(w364, "_Decay.acq") -> (w362:string)
            n164 = property on="Data Directory" class="Path"() -> ("Value"=w361:path)  [unwired: 2 in, 2 out]
            n165 = Build Path(base path=w361, name or relative path=w362) -> (appended path=w360:path)
            n166 = Build Path(base path=w361, name or relative path=w368) -> (appended path=w367:path)
            n167 = Open/Create/Replace File(file path (use dialog)=w360, operation (0:open)=T1."create") -> (refnum out=w366:refnum<file>)  [unwired: 4 in, 2 out]
            n168 = Build Array(w370, w369) -> (w357:dbl[][])
            n169 = Transpose 2D Array(2D array=w357) -> (transposed array=w356:dbl[][])
            n170 = Write to Binary File(file (use dialog)=w366, data=w356, 5:FALSE ("prepend array or string size? (T)")) -> (refnum out=w365:refnum<file>)  [unwired: 3 in, 2 out]
            n171 = call-poly <vilib>:"Write To Spreadsheet File.vi"("format (%.3f)"="%e", "2D data"=w356, "file path (dialog if empty)"=w367) -> ()  [unwired: 5 in, 1 out]
            n172 = Close File(refnum=w365) -> ()  [unwired: 1 in, 2 out]
          }
          frame 6 {
            (unwired) 100000
            w377 = 0.0
            w399 = 10123 items=["Finite Samples"=10178, "Continuous Samples"=10123] ("sample mode")
            w403 = T2 3 items=["no dialog", "OK message", "continue or stop message", "OK message + warnings", "continue/stop + warnings"] ("type of dialog (OK msg:1)")
            w407 = 10123 items=["Finite Samples"=10178, "Continuous Samples"=10123, "Hardware Timed Single Point"=12522] ("sample mode")
            n173 = call-poly <vilib>:"DAQmx Create Virtual Channel.vi"("maximum value"=10.0 ("maximum value 2"), "minimum value"=-10.0 ("minimum value 2"), "physical channels"=tag "Dev1/ao1" ("physical channels 2")) -> ("task out"=w409:refnum<k21>, "error out"=w408:errorcluster)  [unwired: 11 in]
            n174 = call-poly <vilib>:"DAQmx Create Virtual Channel.vi"("maximum value"=10.0 ("Maximum Value 2"), "minimum value"=-10.0 ("Minimum Value 2"), "physical channels"=tag "Dev1/ai0" ("Physical Channel 2")) -> ("task out"=w397:refnum<k21>, "error out"=w398:errorcluster)  [unwired: 11 in]
            n175 = call-poly <vilib>:"DAQmx Timing.vi"("task/channels in"=w397, "sample mode"=w399, "samples per channel"=2, "rate"=5000.0 ("Rate 2"), "error in"=w398) -> ("task out"=w393:refnum<k21>, "error out"=w392:errorcluster)  [unwired: 9 in]
            n176 = call-poly <vilib>:"DAQmx Timing.vi"("task/channels in"=w409, "sample mode"=w407, "rate"=5000, "error in"=w408) -> ("task out"=w406:refnum<k21>, "error out"=w405:errorcluster)  [unwired: 10 in]
            n177 = property class="DAQmx Timing" props=["Sample Clock:Rate"](reference=w393, error in=w392) -> (reference out=w391:refnum<k21>, error out=w390:errorcluster)  [unwired: 1 out]
            n178 = call <vilib>:"DAQmx Start Task.vi"("task/channels in"=w406, "error in"=w405) -> ("task out"=w404:refnum<k21>, "error out"=w386:errorcluster)  [unwired: 12 in]
            n179 = call "Get Terminal Name with Device Prefix.vi"("error in (no error)"=w390, "Local Terminal Name"="ai/StartTrigger" ("terminal"), "task/channels in"=w391) -> ("error out"=w374:errorcluster, "task out"=w375:refnum<k21>)  [unwired: 6 in, 1 out]
            n180 = property on="Waveform Chart" class="WFChart (strict)"("Visible"=TRUE) -> ()  [unwired: 2 in, 2 out]
            n181 = call <vilib>:"DAQmx Start Task.vi"("task/channels in"=w375, "error in"=w374) -> ("task out"=w384:refnum<k21>, "error out"=w388:errorcluster)  [unwired: 12 in]
            n182 = Initialize Array(w377, w377) -> ()  [unwired: 1 out]
            n183 = while {
              tunnel: w404 -> [w435]
              tunnel: w388 -> [w434]
              tunnel: w386 -> [w433]
              tunnel: ["Analog Ouyput 1"] -> w385
              tunnel: w384 -> [w432]
              tunnel: [w431] -> w383
              tunnel: [w430] -> w382
              tunnel: [w429] -> w380
              tunnel: [w423] -> w378
              stop <- w420 stop-if-true
              n184 = call-poly <vilib>:"DAQmx Read.vi"("task/channels in"=w432, "error in"=w434) -> ("task out"=w423:refnum<k21>, "data"=w418:dbl, "error out"=w429:errorcluster)  [unwired: 11 in]
              "Waveform Chart" <- w418
              n185 = call-poly <vilib>:"DAQmx Write.vi"("task/channels in"=w435, "data"="Analog Ouyput 1", "timeout"=0.1 ("Wirite Timeout"), "error in"=w433) -> ("task out"=w431:refnum<k21>, "error out"=w430:errorcluster)  [unwired: 9 in, 1 out]
              n186 = local read "Manual Z"() -> (w417:bool)
              n187 = local read "Sweep Bias"() -> (w421:bool)
              n188 = local read "Save IV"() -> (w419:bool)
              n189 = Build Array("Analog Ouyput 1") -> (w427:dbl[])
              n190 = Build Array(w418) -> (w426:dbl[])
              n191 = Build Array(w426, w427) -> (w425:dbl[][])
              n192 = Not(x=w417) -> (.not. x?=w422:bool)
              n193 = Transpose 2D Array(2D array=w425) -> ()  [unwired: 1 out]
              n194 = Compound Arithmetic op=OR(w419, w421, w422) -> (w420:bool)
            }
            n195 = call <vilib>:"DAQmx Clear Task.vi"("task in"=w383, "error in"=w382) -> ("error out"=w381:errorcluster)  [unwired: 13 in]
            n196 = call <vilib>:"DAQmx Clear Task.vi"("task in"=w378, "error in"=w380) -> ("error out"=w379:errorcluster)  [unwired: 13 in]
            n197 = Merge Errors(w379, w381) -> (w387:errorcluster)
            n198 = call <vilib>:"General Error Handler.vi"("type of dialog (OK msg:1)"=w403, "error in (no error)"=w387) -> ()  [unwired: 9 in, 5 out]
          }
          frame 7 {
            w439 = 0.0
            w460 = T2 3 items=["no dialog", "OK message", "continue or stop message", "OK message + warnings", "continue/stop + warnings"] ("type of dialog (OK msg:1)")
            w475 = 10123 items=["Finite Samples"=10178, "Continuous Samples"=10123] ("sample mode")
            w469 = 10123 items=["Finite Samples"=10178, "Continuous Samples"=10123] ("sample mode")
            n199 = call-poly <vilib>:"DAQmx Create Virtual Channel.vi"("maximum value"=10.0 ("maximum value 2"), "minimum value"=-10.0 ("minimum value 2"), "physical channels"=tag "Dev1/ao1" ("physical channels 2")) -> ("task out"=w476:refnum<k21>, "error out"=w477:errorcluster)  [unwired: 11 in]
            n200 = call-poly <vilib>:"DAQmx Create Virtual Channel.vi"("maximum value"=10.0 ("Maximum Value 2"), "minimum value"=-10.0 ("Minimum Value 2"), "physical channels"=tag "Dev1/ai0" ("Physical Channel 2")) -> ("task out"=w471:refnum<k21>, "error out"=w470:errorcluster)  [unwired: 11 in]
            n201 = call-poly <vilib>:"DAQmx Timing.vi"("task/channels in"=w476, "sample mode"=w475, "rate"=10000.0 ("rate 2"), "error in"=w477) -> ("task out"=w484:refnum<k21>, "error out"=w485:errorcluster)  [unwired: 10 in]
            n202 = call-poly <vilib>:"DAQmx Timing.vi"("task/channels in"=w471, "sample mode"=w469, "rate"=10000.0 ("Rate 2"), "error in"=w470) -> ("task out"=w487:refnum<k21>, "error out"=w488:errorcluster)  [unwired: 10 in]
            n203 = property class="DAQmx Timing" props=["Sample Clock:Rate"](reference=w484, error in=w485) -> (reference out=w483:refnum<k21>, error out=w486:errorcluster)  [unwired: 1 out]
            n204 = property class="DAQmx Timing" props=["Sample Clock:Rate"](reference=w487, error in=w488) -> (reference out=w489:refnum<k21>, error out=w490:errorcluster)  [unwired: 1 out]
            n205 = call "Get Terminal Name with Device Prefix.vi"("error in (no error)"=w490, "Local Terminal Name"="ai/StartTrigger" ("terminal"), "task/channels in"=w489) -> ("error out"=w458:errorcluster, "Terminal Name with Device Prefix"=w482:tag, "task out"=w456:refnum<k21>)  [unwired: 6 in]
            n206 = call-poly <vilib>:"DAQmx Trigger.vi"("task/channels in"=w483, "source"=w482, "error in"=w486) -> ("task out"=w451:refnum<k21>, "error out"=w448:errorcluster)  [unwired: 11 in]
            n207 = Initialize Array(0.0, "Step Length") -> (w454:dbl[])
            n208 = call <vilib>:"DAQmx Start Task.vi"("task/channels in"=w456, "error in"=w458) -> ("task out"=w455:refnum<k21>, "error out"=w457:errorcluster)  [unwired: 12 in]
            n209 = call <vilib>:"DAQmx Start Task.vi"("task/channels in"=w451, "error in"=w448) -> ("task out"=w450:refnum<k21>, "error out"=w449:errorcluster)  [unwired: 12 in]
            n210 = Initialize Array(w439, w439) -> (w438:dbl[])
            n211 = while {
              tunnel: w455 -> [w511]
              tunnel: w457 -> [w510]
              tunnel: w450 -> [w509]
              tunnel: w449 -> [w508]
              tunnel: [w507] -> w466
              tunnel: [w506] -> w465
              tunnel: [w505] -> w463
              tunnel: [w504] -> w461
              shift-right: [w502] -> _
              shift-left: w454 -> [w503]
              tunnel: w446 -> [w500]
              shift-right: [w499] -> _
              shift-left: 1 -> [w498]
              shift-right: [w497] -> w442
              shift-left: w447 -> [w501]
              shift-right: [w495] -> w441
              shift-left: w438 -> [w496]
              shift-right: [w493] -> w440
              shift-left: w438 -> [w494]
              tunnel: [w491] -> w437
              stop <- w491 stop-if-true
              n212 = stacked-sequence {
                seq-local: [w513 _] -> [_ w553]
                tunnel: w511 -> [w544 _]
                tunnel: w510 -> [w543 _]
                tunnel: w509 -> [_ w561]
                tunnel: w508 -> [_ w560]
                tunnel: [w541 _] -> w507
                tunnel: [w542 _] -> w506
                tunnel: [_ w558] -> w505
                tunnel: [_ w559] -> w504
                tunnel: w503 -> [w538 w545]
                tunnel: [w521 _] -> w502
                tunnel: [w514 _] -> w491
                tunnel: w501 -> [_ w557]
                tunnel: w500 -> [_ w556]
                tunnel: [_ w555] -> w499
                tunnel: w498 -> [w530 w554]
                tunnel: "Ramp Rate" -> [_ w552]
                tunnel: [_ w550] -> _
                tunnel: [_ w550] -> w497
                tunnel: w496 -> [_ w549]
                tunnel: [_ w548] -> w495
                tunnel: w494 -> [_ w547]
                tunnel: [_ w546] -> w493
                frame #0 {
                  n213 = call-poly <vilib>:"DAQmx Read.vi"("task/channels in"=w544, "error in"=w543) -> ("task out"=w541:refnum<k21>, "data"=w512:dbl, "error out"=w542:errorcluster)  [unwired: 11 in]
                  n214 = Absolute Value(x=w512) -> (abs(x)=w513:dbl)
                  n215 = Insert Into Array(array=w538, index=0, new element=w513) -> (w539:dbl[])
                  n216 = local write "Waveform Chart"(w513) -> ()
                  n217 = Delete From Array(array=w539, length=1) -> (array with subset deleted=w521:dbl[])  [unwired: 1 in, 1 out]
                  n218 = Array Size(array=w521) -> (size(s)=w531:i32)
                  n219 = Decrement(x=w531) -> (x-1=w522:i32)
                  n220 = Index Array(array=w521, index=w522) -> (element=w524:dbl)
                  "element" <- w524
                  n221 = Index Array(array=w521, index=0) -> (element=w526:dbl)
                  n222 = Less?(x=w521, y="Step Max") -> (x < y?=w536:bool[])
                  n223 = Greater?(x=w521, y="Step Min") -> (0:w535:bool[])
                  n224 = Greater?(x="Step Min", y=w524) -> ()  [unwired: 1 out]
                  n225 = And Array Elements(Boolean array=w536) -> (logical AND=w520:bool)
                  n226 = And Array Elements(Boolean array=w535) -> (logical AND=w519:bool)
                  n227 = Less?(x="Step Max", y=w526) -> ()  [unwired: 1 out]
                  n228 = local read "Tapping"() -> (w516:bool)
                  n229 = And(x=w520, y=w519) -> (x .and. y?=w534:bool)
                  n230 = Equal?(x=w530, y=1) -> (x = y?=w528:bool)
                  n231 = Equal?(x=w530, y=2) -> (x = y?=w527:bool)
                  n232 = Or(x=w528, y=w527) -> (x .or. y?=w518:bool)
                  n233 = Not(x=w516) -> (.not. x?=w515:bool)
                  n234 = Compound Arithmetic op=AND(w534, w518) -> (w517:bool)
                  "Tapping Stop" <- w517
                  n235 = Or(x=w517, y=w515) -> (x .or. y?=w514:bool)
                }
                frame #1 {
                  n236 = case shown="1, Default" w554 {
                    tunnel: [w569 w592 w613 w639] -> w550
                    tunnel: w557 -> [w582 w594 w624 w636]
                    tunnel: [w577 w593 w618 w635] -> w555
                    tunnel: w553 -> [w568 _ w623 _]
                    tunnel: w552 -> [w583 w597 w625 w634]
                    tunnel: w549 -> [w573 w591 w612 _]
                    tunnel: [w575 w591 w612 w632] -> w548
                    tunnel: w547 -> [w567 w590 w611 _]
                    tunnel: [w574 w590 w611 w632] -> w546
                    tunnel: w545 -> [w566 _ _ _]
                    frame 1, Default {
                      w571 = -10
                      # "Breaking the contact"
                      n237 = Divide(x=w583, y=15.13) -> (x/y=w587:dbl)
                      n238 = Array Subset(array=w566, index=0, length=10) -> (w563:dbl[])
                      n239 = Divide(x=20, y=32768) -> (x/y=w584:dbl)
                      n240 = call-poly <vilib>:"Mean.vi"("X"=w563) -> ("mean"=w562:dbl)  [unwired: 1 out]
                      "mean" <- w562
                      n241 = Multiply(x=w584, y=w587) -> (x*y=w589:dbl)
                      n242 = Subtract(x=w582, y=w589) -> (x-y=w570:dbl)
                      n243 = Less?(x=w562, y="Min Current") -> (x < y?=w580:bool)
                      n244 = Select(t=2, s=w580, f=1) -> (s? t:f=w577:i32)
                      n245 = Build Array (concatenate)(w570, w573) -> (w575:dbl[])
                      n246 = Build Array (concatenate)(w568, w567) -> (w574:dbl[])
                      n247 = Less?(x=w570, y=w571) -> (x < y?=w572:bool)
                      n248 = local write "Contact Cycles"(0) -> ()
                      n249 = Select(t=w571, s=w572, f=w570) -> (s? t:f=w569:dbl)
                    }
                    frame 2 {
                      w609 = 10
                      # "Break contact cycles after current = 0"
                      n250 = Divide(x=w597, y=15.13) -> (x/y=w605:dbl)
                      n251 = local read "Contact Cycles"() -> (w596:i32)
                      n252 = Divide(x=20, y=32768) -> (x/y=w598:dbl)
                      n253 = Multiply(x=w598, y=w605) -> (x*y=w607:dbl)
                      n254 = Subtract(x=w594, y=w607) -> (x-y=w599:dbl)
                      n255 = Increment(x=w596) -> (x+1=w595:i32)
                      n256 = Less?(x=w599, y=w609) -> (x < y?=w608:bool)
                      n257 = Select(t=w599, s=w608, f=w609) -> (s? t:f=w592:dbl)
                      n258 = Less Or Equal?(x="Break Contact", y=w595) -> (x <= y?=w602:bool)
                      n259 = local write "Contact Cycles"(w595) -> ()
                      n260 = Select(t=3, s=w602, f=2) -> (s? t:f=w593:i32)
                    }
                    frame 3 {
                      w616 = 10
                      # "Making contact"
                      n261 = Divide(x=w625, y=15.13) -> (x/y=w629:dbl)
                      n262 = Divide(x=20, y=32768) -> (x/y=w626:dbl)
                      n263 = Multiply(x=w626, y=w629) -> (x*y=w631:dbl)
                      n264 = Add(x=w624, y=w631) -> (x+y=w614:dbl)
                      n265 = Greater?(x=w623, y="Max Current") -> (0:w621:bool)
                      n266 = Select(t=4, s=w621, f=3) -> (s? t:f=w618:i32)
                      n267 = local write "Contact Cycles"(0) -> ()
                      n268 = Less?(x=w614, y=w616) -> (x < y?=w615:bool)
                      n269 = Select(t=w614, s=w615, f=w616) -> (s? t:f=w613:dbl)
                    }
                    frame 4 {
                      w633 = 0.0
                      w651 = 10
                      # "Make contact cycles after current saturation"
                      n270 = Divide(x=w634, y=15.13) -> (x/y=w647:dbl)
                      n271 = local read "Contact Cycles"() -> (w641:i32)
                      n272 = Divide(x=20, y=32768) -> (x/y=w637:dbl)
                      n273 = Multiply(x=w637, y=w647) -> (x*y=w649:dbl)
                      n274 = Add(x=w636, y=w649) -> (x+y=w638:dbl)
                      n275 = Increment(x=w641) -> (x+1=w640:i32)
                      n276 = Less?(x=w638, y=w651) -> (x < y?=w650:bool)
                      n277 = Select(t=w638, s=w650, f=w651) -> (s? t:f=w639:dbl)
                      n278 = Less Or Equal?(x="Make Contact", y=w640) -> (x <= y?=w644:bool)
                      n279 = local write "Contact Cycles"(w640) -> ()
                      n280 = Initialize Array(w633, w633) -> (w632:dbl[])
                      n281 = Select(t=1, s=w644, f=4) -> (s? t:f=w635:i32)
                    }
                  }
                  n282 = local write "Analog Ouyput 1"(w550) -> ()
                  n283 = Build Array(w556, w550) -> ()  [unwired: 1 out]
                  n284 = call-poly <vilib>:"DAQmx Write.vi"("task/channels in"=w561, "auto start"=TRUE, "data"=w550, "error in"=w560) -> ("task out"=w559:refnum<k21>, "error out"=w558:errorcluster)  [unwired: 9 in, 1 out]
                }
              }
              "Case" <- w499
            }
            n285 = call <vilib>:"DAQmx Clear Task.vi"("task in"=w461, "error in"=w463) -> ("error out"=w462:errorcluster)  [unwired: 13 in]
            n286 = Not(x=w437) -> (.not. x?=w436:bool)
            n287 = call <vilib>:"DAQmx Clear Task.vi"("task in"=w466, "error in"=w465) -> ("error out"=w464:errorcluster)  [unwired: 13 in]
            n288 = local write "Tapping"(w436) -> ()
            n289 = Merge Errors(w464, w462) -> (w459:errorcluster)
            n290 = call <vilib>:"General Error Handler.vi"("type of dialog (OK msg:1)"=w460, "error in (no error)"=w459) -> ()  [unwired: 9 in, 5 out]
          }
          frame 8 {
            w658 = 0.0
            w672 = T2 3 items=["no dialog", "OK message", "continue or stop message", "OK message + warnings", "continue/stop + warnings"] ("type of dialog (OK msg:1)")
            w685 = 10123 items=["Finite Samples"=10178, "Continuous Samples"=10123] ("sample mode")
            w679 = 10123 items=["Finite Samples"=10178, "Continuous Samples"=10123] ("sample mode")
            n291 = call-poly <vilib>:"DAQmx Create Virtual Channel.vi"("maximum value"=10.0 ("maximum value 2"), "minimum value"=-10.0 ("minimum value 2"), "physical channels"=tag "Dev1/ao0:1" ("physical channels 2")) -> ("task out"=w686:refnum<k21>, "error out"=w687:errorcluster)  [unwired: 11 in]
            n292 = call-poly <vilib>:"DAQmx Create Virtual Channel.vi"("maximum value"=10.0 ("Maximum Value 2"), "minimum value"=-10.0 ("Minimum Value 2"), "physical channels"=tag "Dev1/ai0" ("Physical Channel 2")) -> ("task out"=w681:refnum<k21>, "error out"=w680:errorcluster)  [unwired: 11 in]
            n293 = call-poly <vilib>:"DAQmx Timing.vi"("task/channels in"=w686, "sample mode"=w685, "rate"=10000.0 ("rate 2"), "error in"=w687) -> ("task out"=w694:refnum<k21>, "error out"=w695:errorcluster)  [unwired: 10 in]
            n294 = call-poly <vilib>:"DAQmx Timing.vi"("task/channels in"=w681, "sample mode"=w679, "rate"=10000.0 ("Rate 2"), "error in"=w680) -> ("task out"=w697:refnum<k21>, "error out"=w698:errorcluster)  [unwired: 10 in]
            n295 = property class="DAQmx Timing" props=["Sample Clock:Rate"](reference=w694, error in=w695) -> (reference out=w693:refnum<k21>, error out=w696:errorcluster)  [unwired: 1 out]
            n296 = property class="DAQmx Timing" props=["Sample Clock:Rate"](reference=w697, error in=w698) -> (reference out=w699:refnum<k21>, error out=w700:errorcluster)  [unwired: 1 out]
            n297 = call "Get Terminal Name with Device Prefix.vi"("error in (no error)"=w700, "Local Terminal Name"="ai/StartTrigger" ("terminal"), "task/channels in"=w699) -> ("error out"=w670:errorcluster, "Terminal Name with Device Prefix"=w692:tag, "task out"=w668:refnum<k21>)  [unwired: 6 in]
            n298 = call-poly <vilib>:"DAQmx Trigger.vi"("task/channels in"=w693, "source"=w692, "error in"=w696) -> ("task out"=w666:refnum<k21>, "error out"=w663:errorcluster)  [unwired: 11 in]
            n299 = call <vilib>:"DAQmx Start Task.vi"("task/channels in"=w668, "error in"=w670) -> ("task out"=w667:refnum<k21>, "error out"=w669:errorcluster)  [unwired: 12 in]
            n300 = call <vilib>:"DAQmx Start Task.vi"("task/channels in"=w666, "error in"=w663) -> ("task out"=w665:refnum<k21>, "error out"=w664:errorcluster)  [unwired: 12 in]
            n301 = Initialize Array(w658, w658) -> ()  [unwired: 1 out]
            n302 = while {
              tunnel: w667 -> [w735]
              tunnel: w669 -> [w734]
              tunnel: w665 -> [w724]
              tunnel: w664 -> [w723]
              tunnel: [w733] -> w676
              tunnel: [w732] -> w675
              shift-right: [w709] -> w659
              shift-left: w662 -> [w714]
              tunnel: [w722] -> w657
              tunnel: [w721] -> w656
              tunnel: w653 -> [w705]
              i -> [w720]
              stop <- w710 stop-if-true
              w718 = 5e-05
              n303 = Absolute Value(x="Setpoint") -> (abs(x)=w701:dbl)
              n304 = call-poly <vilib>:"DAQmx Read.vi"("task/channels in"=w735, "error in"=w734) -> ("task out"=w733:refnum<k21>, "data"=w704:dbl, "error out"=w732:errorcluster)  [unwired: 11 in]
              n305 = Absolute Value(x=w704) -> (abs(x)=w703:dbl)
              n306 = local read "Bias Offset Correct"() -> (w706:dbl)
              n307 = Bundle("Proportional Gain"="Proportional Gain", "Integral Gain"="Integral Gain", "Differential Gain"="Differential Gain") -> (w725:T3)  [unwired: 1 in]
              n308 = local write "Waveform Chart"(w704) -> ()
              n309 = Bundle(10, -10) -> (w729:cluster{i32, i32})  [unwired: 1 in]
              n310 = call-poly "PID.vi"("output range"=w729, "dt (s)"=w718, "PID gains"=w725, "process variable"=w703, "setpoint"=w701) -> ("output"=w717:dbl)  [unwired: 5 in, 1 out]
              n311 = Add(x=w705, y=w706) -> (x+y=w707:dbl)
              n312 = Less?(x=w720, y=1000) -> (x < y?=w715:bool)
              n313 = call-poly "PID Output Rate Limiter.vi"("reinitialize? (F)"=w715, "dt (s)"=w718, "output rate (EGU/min)"="Piezo Delta rate", "initial output"=w714, "input (controller output)"=w717) -> ("output"=w709:dbl)  [unwired: 3 in, 1 out]
              n314 = local write "Analog Ouyput 1"(w709) -> ()
              n315 = Build Array(w707, w709) -> (w708:dbl[])
              n316 = local read "Sweep Bias"() -> (w713:bool)
              n317 = local read "PID"() -> (w711:bool)
              n318 = call-poly <vilib>:"DAQmx Write.vi"("task/channels in"=w724, "data"=w708, "error in"=w723) -> ("task out"=w722:refnum<k21>, "error out"=w721:errorcluster)  [unwired: 10 in, 1 out]
              n319 = Not(x=w711) -> (.not. x?=w712:bool)
              n320 = Compound Arithmetic op=OR(w713, w712) -> (w710:bool)
            }
            n321 = call <vilib>:"DAQmx Clear Task.vi"("task in"=w657, "error in"=w656) -> ("error out"=w673:errorcluster)  [unwired: 13 in]
            n322 = call <vilib>:"DAQmx Clear Task.vi"("task in"=w676, "error in"=w675) -> ("error out"=w674:errorcluster)  [unwired: 13 in]
            n323 = Merge Errors(w674, w673) -> (w671:errorcluster)
            n324 = call <vilib>:"General Error Handler.vi"("type of dialog (OK msg:1)"=w672, "error in (no error)"=w671) -> ()  [unwired: 9 in, 5 out]
          }
        }
      }
    }
  }
